vi "Create JSON Schema.vi"(5 "JSON Schema Description":string, 6 "Write to File? [F]":bool, 7 "JSON Schema Title":string, 8 "error in (no error)":errorcluster, 9 "LV Object":variant, 11 "JSON Schema in":string) -> (0 "error out":errorcluster)   [LabVIEW 2019, in "JSON-Schema.lvlib"]
doc: "Generates a JSON Schema for <b>LV object</b> and merges with an existing (optional) <b>JSON Schema in</b>.\n\n<b>Write to File?</b> write the generated JSON Schema to an existing typedef control file."
uses:
  JSON-Schema.lvlib
panel:
  out "JSON Schema out":string
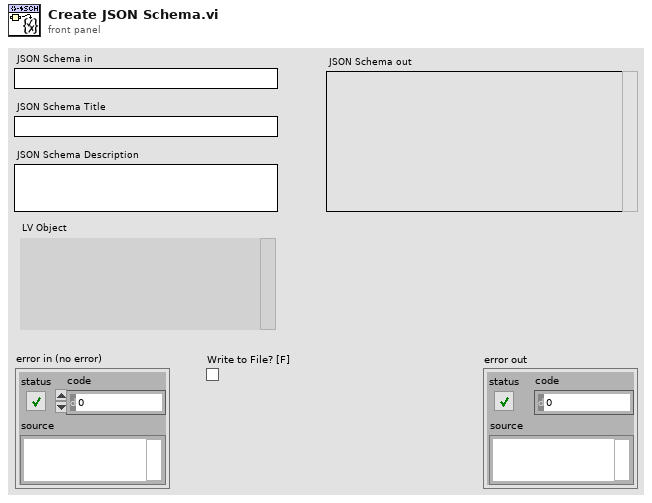
[diagram p1: front panel]
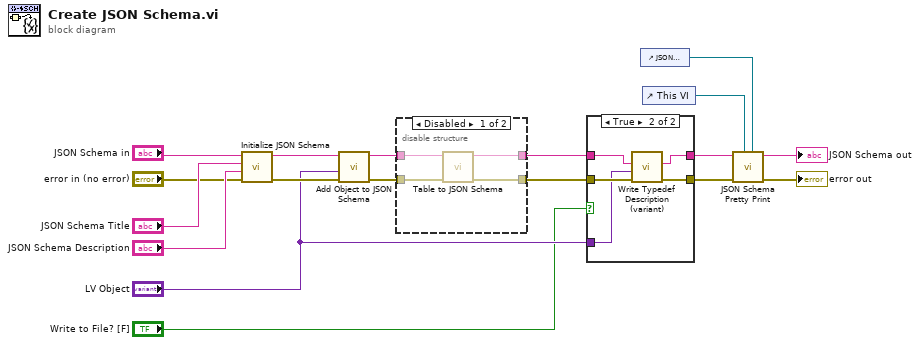
[diagram p0: block diagram]
diagram:
  n1 = call "Initialize JSON Schema.vi"("error in (no error)"="error in (no error)", "Description"="JSON Schema Description", "Title"="JSON Schema Title", "JSON Schema in"="JSON Schema in") -> ("error out"=w13:errorcluster, "JSON Schema out"=w15:string)  [unwired: 6 in]
  n2 = call "Add Object to JSON Schema.vi"("error in (no error)"=w13, "Object"="LV Object", "JSON Schema in"=w15) -> ("error out"=w12:errorcluster, "JSON Schema out"=w14:string)  [unwired: 7 in]
  n3 = disable-structure shown="Disabled" {
    disable-tunnel: w14 -> [w22 w23]
    disable-tunnel: w12 -> [w21 _]
    disable-tunnel: [w20 w23] -> w10
    disable-tunnel: [w19 _] -> w11
    frame Disabled {
      n4 = call "Table to JSON Schema.vi"("error in (no error)"=w21, "JSON Schema in"=w22) -> ("error out"=w19:errorcluster, "JSON Schema out"=w20:string)  [unwired: 8 in]
    }
    frame Enabled {
    }
  }
  n5 = case shown="True" "Write to File? [F]" {
    tunnel: w11 -> [w24 w30]
    tunnel: w10 -> [w25 w27]
    tunnel: "LV Object" -> [_ w29]
    tunnel: [w24 w28] -> w4
    tunnel: [w25 w26] -> w6
    frame False {
    }
    frame True {
      n6 = call "Write Typedef Description (variant).vi"("error in (no error)"=w30, "variant"=w29, "VI Description in"=w27) -> ("error out"=w28:errorcluster, "VI Description out"=w26:string)  [unwired: 7 in]
    }
  }
  n7 = control-ref of="JSON Schema out"() -> (w2:refnum<vi>)
  n8 = control-ref of="This VI"() -> (w1:refnum<vi>)
  n9 = call "JSON Schema Pretty Print.vi"("String Control"=w2, "reference"=w1, "error in (no error)"=w4, "<JSON> in"=w6) -> ("error out"=→"error out":errorcluster, "<JSON> out"=→"JSON Schema out":string)  [unwired: 6 in]
